vi "MetaData Channel.vi"(8 "error in (no error)":errorcluster, 11 "Node Ptr":T5 format="%.0x") -> (0 "error out":errorcluster)   [LabVIEW 2019, in "Instrument Addon System Explorer.lvlib"]
uses:
  Instrument Addon System Explorer.lvlib
  <vilib>/NI VeriStand/Custom Device API/Custom Device Item Ref.ctl
  Addon Shared/Types/Protocol Data Type.ctl
  Addon Shared/Types/Metadata Channel Type.ctl
  Addon Shared/Types/Type Cast Type.ctl
  Addon Shared/Types/Endian.ctl
  Addon Shared/Types/FG Control.ctl
  Addon Shared/SubVIs/Constants.vi
  <vilib>/NI VeriStand/Custom Device API/NI VeriStand - Get Item Property.vi
  <vilib>/NI VeriStand/Custom Device API/Get Item Property (U32).vi
  <vilib>/NI VeriStand/Custom Device API/Get Item Property (String Array).vi
  <vilib>/NI VeriStand/Custom Device API/Get Item Property (String).vi
  <vilib>/NI VeriStand/Custom Device API/NI VeriStand - Set Item Property.vi
  <vilib>/NI VeriStand/Custom Device API/Set Item Property (U32).vi
  <vilib>/NI VeriStand/Custom Device API/Set Item Property (String Array).vi
  Addon Shared/SubVIs/Set Channel Value Table.vi
  <vilib>/NI VeriStand/Custom Device API/Set Item Property (String).vi
  <vilib>/NI VeriStand/Custom Device API/Custom Device API.lvlib
  Addon Shared/Instrument Addon Shared.lvlib
  APIs/Scripting API/Instrument Addon Scripting API.lvlib
panel:
  in  "Delimiter":string=","
  in  "Reset":bool
  in  "Create":bool
  in  "Elements":u32
  in  "Units":string
  in  "Default Value":dbl
  out "Channel Type (Tab)":enum32{"List", "Format", "Type Cast"}(tab)
  in  "Remove":bool
  in  "Add":bool
  in  "Enumerated List":i32(listbox)
  in  "Test Value":dbl
  in  "Format String":string="%.3g"
  out "Validated String":string
  in  "Endian":T1=enum."Little"
  in  "Type":T2
  in  "Channel Type":T3
  out "Data Type":T4
  in  "Header 2":cluster{"Section Name":string}={"Section Name"="MetaData Format Settings"}
  in  "SHDocVw.IWebBrowser":refnum<k7>(container)
  in  "Header":cluster{"Section Name":string}={"Section Name"="MetaData Settings"}
  in  "Description":string
  in  "Name":string
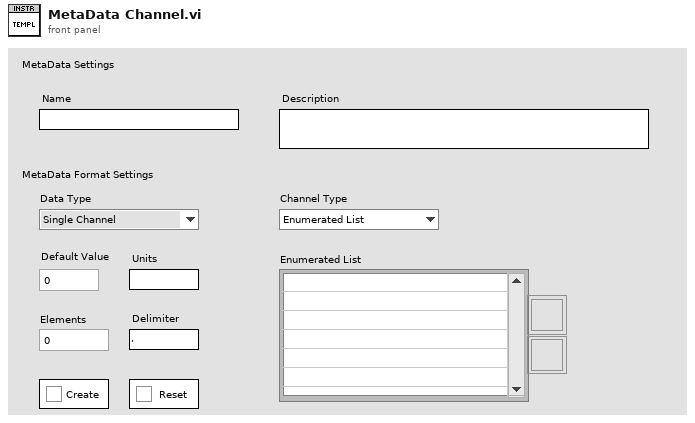
[diagram p1: front panel]
types:
  T1 = typedef "Instrument Addon Shared.lvlib/Endian.ctl" = enum16{"Native", "Little", "Big"}
  T2 = typedef "Instrument Addon Shared.lvlib/Type Cast Type.ctl" = enum16{"DBL", "SGL", "U64", "U32", "U16", "U8", "I64", "I32", "I16", "I8"}
  T3 = typedef "Instrument Addon Shared.lvlib/Metadata Channel Type.ctl" = enum16{"Enumerated List", "Format", "Type Cast"}
  T4 = typedef "Instrument Addon Shared.lvlib/Protocol Data Type.ctl" = enum16{"Single Channel", "Array"}
  T5 = typedef "Custom Device API.lvlib/Custom Device Item Ref.ctl" = u64
  T6 = typedef "Instrument Addon Shared.lvlib/FG Control.ctl" = enum16{"Get", "Set"}
  T7 = typedef "Custom Device API.lvlib/Custom Device Item Info.ctl" = cluster{"Name":string, "Is Channel":bool, "GUID":string, "Is Waveform":bool}
  T8 = typedef "Instrument Addon Shared.lvlib/MetaData Parameters.ctl" = cluster{"Data Type":T4, "Channel Type":T3, "List":string[], "Format String":string, "Type":T2, "Delimiter":string, "Endian":T1}
  T9 = typedef "Custom Device API.lvlib/Custom Device Channel.ctl" = cluster{"Type":T10, "Units":string, "Default Value":dbl, "Faultable":bool, "Scalable":bool}
  T10 = typedef "Custom Device API.lvlib/Custom Device Channel Type.ctl" = enum16{"Input", "Output"}
  T11 = typedef "Custom Device API.lvlib/Custom Device Commands.ctl" = enum16{"Default", "Item renamed", "Shutdown", "Dynamic button pressed"}
  T12 = typedef "Instrument Addon Scripting API.lvlib/Array Element.ctl" = cluster{"Name":string, "Default Value":dbl, "Units":string}
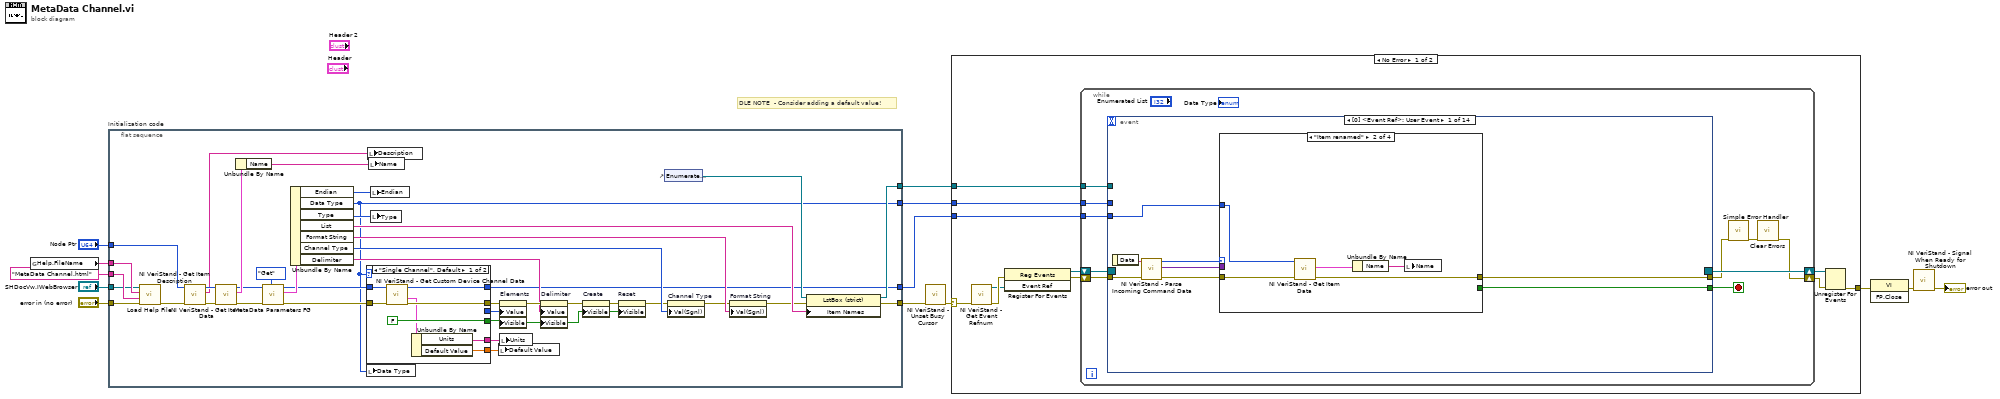
[diagram p0: block diagram]
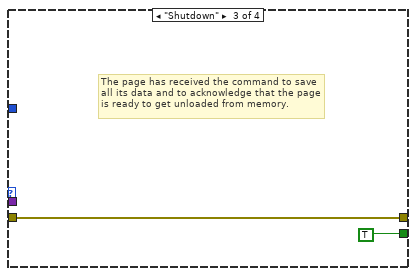
[diagram p3: hidden frame]
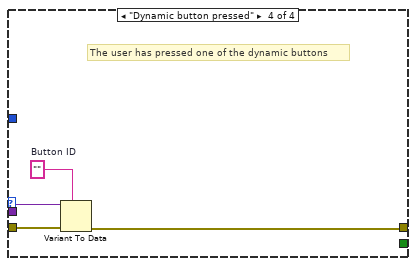
[diagram p4: hidden frame]
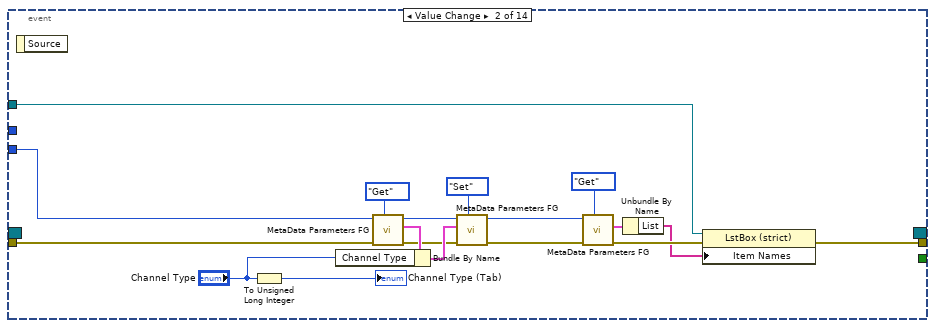
[diagram p5: hidden frame]
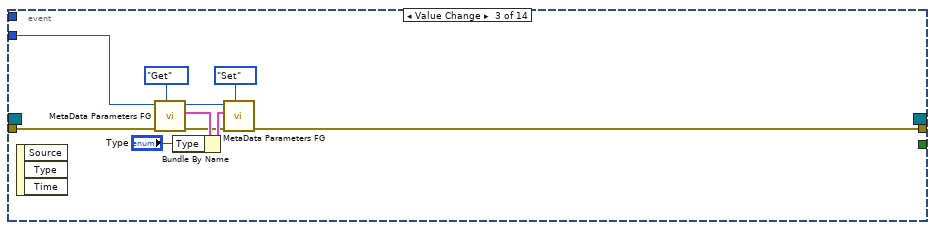
[diagram p6: hidden frame]
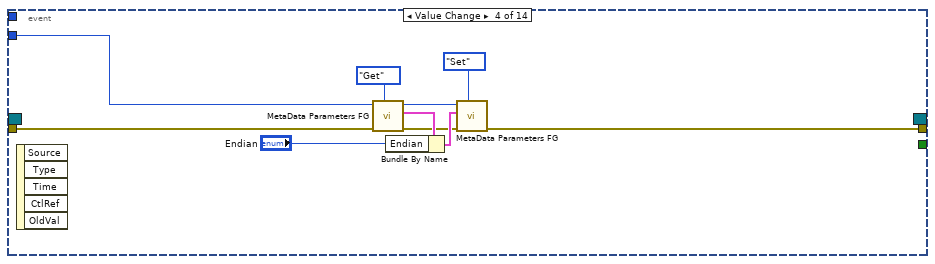
[diagram p7: hidden frame]
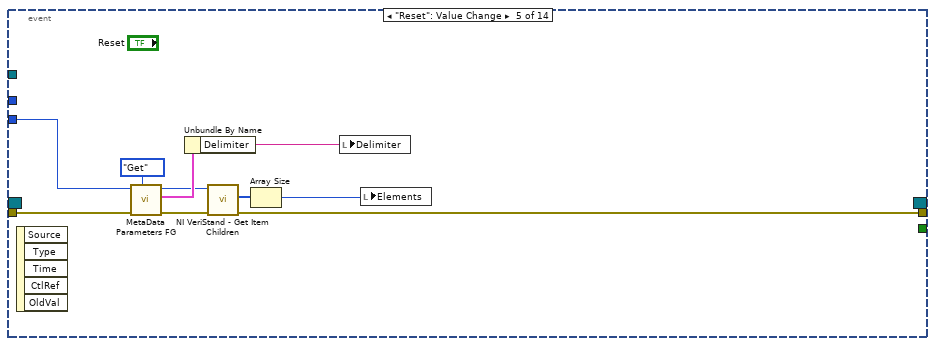
[diagram p8: hidden frame]
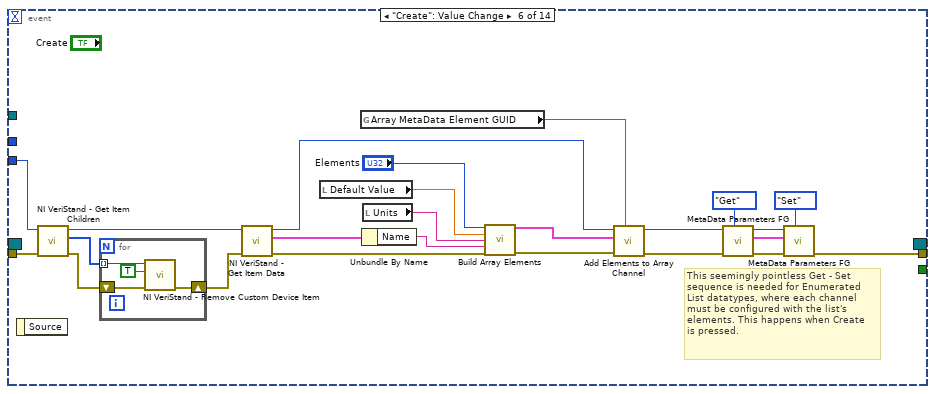
[diagram p9: hidden frame]
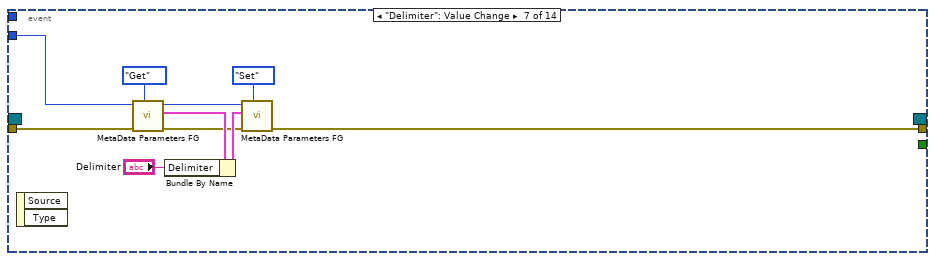
[diagram p10: hidden frame]
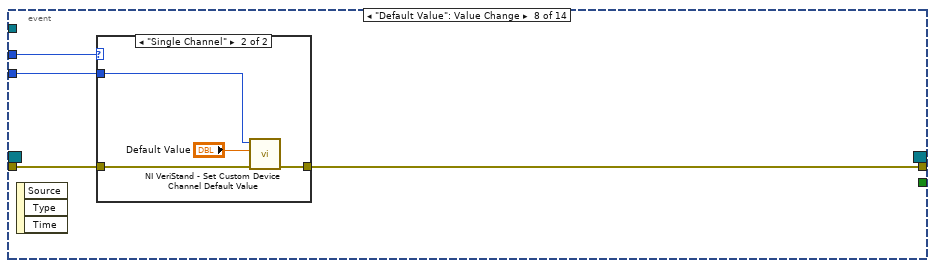
[diagram p11: hidden frame]
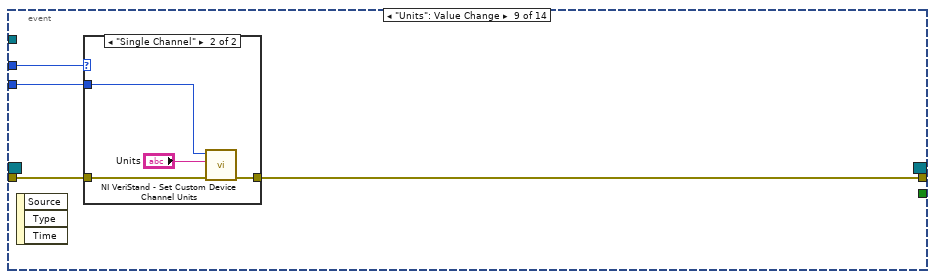
[diagram p13: hidden frame]
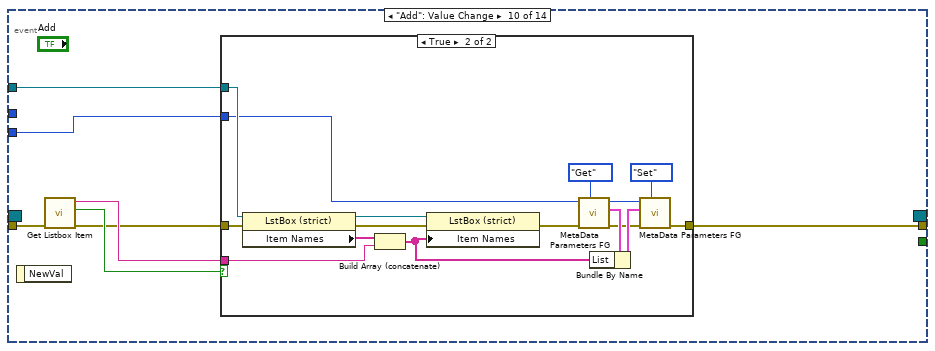
[diagram p15: hidden frame]
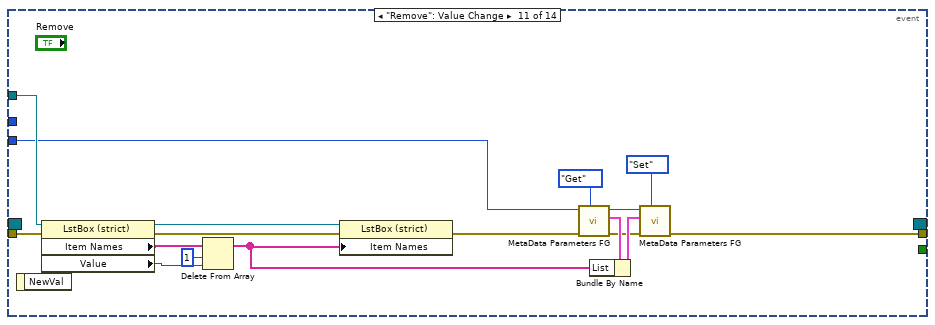
[diagram p17: hidden frame]
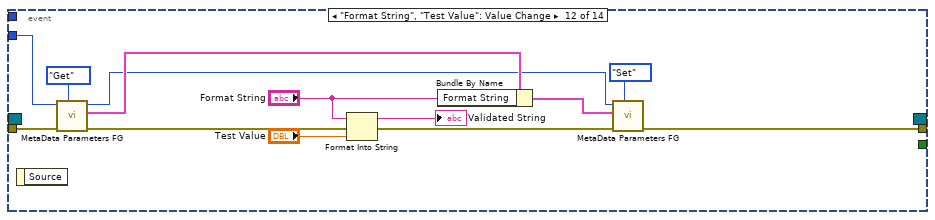
[diagram p18: hidden frame]
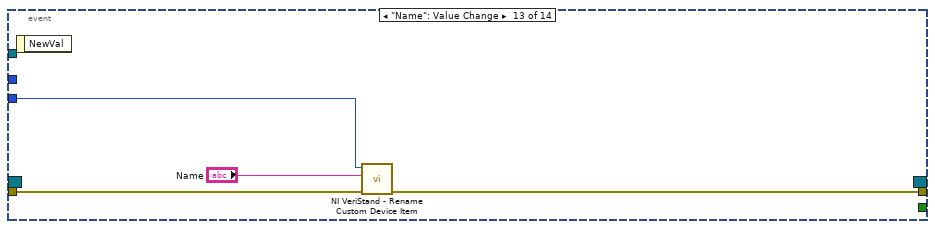
[diagram p19: hidden frame]
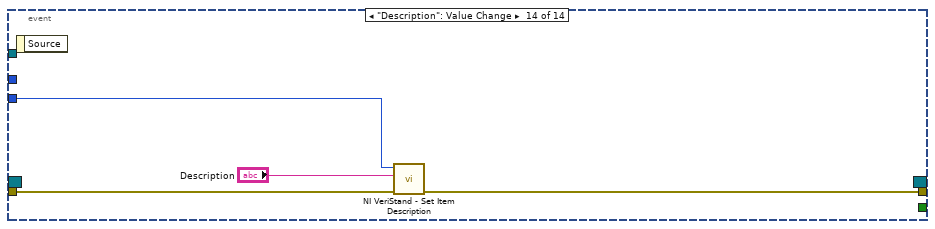
[diagram p20: hidden frame]
diagram:
  # "DLE NOTE  - Consider adding a default value!"
  n1 = global read "Constants.vi" "Help.FileName"() -> (w1:string)
  n2 = flat-sequence "Initialization code" {
    tunnel: "error in (no error)" -> [w47]
    tunnel: "Node Ptr" -> [w32]
    tunnel: [w36] -> w9
    tunnel: [w20] -> w3
    tunnel: w1 -> [w46]
    tunnel: "MetaData Channel.html" ("HTML File") -> [w45]
    tunnel: "SHDocVw.IWebBrowser" -> [w44]
    tunnel: [w34] -> w4
    tunnel: [w17] -> w2
    frame #0 {
      n3 = call "Load Help File.vi"("error in (no error)"=w47, "HTML File"=w45, "Main CHM File"=w46, "SHDocVw.IWebBrowser2"=w44) -> ("error out"=w33:errorcluster)  [unwired: 7 in]
      n4 = call <vilib>:"NI VeriStand - Get Item Description.vi"("error in (no error)"=w33, "Item Ref in"=w32) -> ("error out"=w50:errorcluster, "Description"=w51:string, "Item Ref out"=w52:T5)  [unwired: 7 out]
      n5 = call <vilib>:"NI VeriStand - Get Item Data.vi"("error in (no error)"=w50, "Item Ref in"=w52) -> ("error out"=w25:errorcluster, "Item Info"=w49:T7, "Item Ref out"=w24:T5)  [unwired: 7 out]
      n6 = Unbundle By Name(w49) -> ("Name"=w48:string)
      n7 = call "MetaData Parameters FG.vi"("Action"=FG_Control."Get", "error in (no error)"=w25, "Item Ref in"=w24) -> ("error out"=w23:errorcluster, "MetaData Parameters"=w42:T8, "Item Ref out"=w22:T5)  [unwired: 6 in]
      n8 = Unbundle By Name(w42) -> ("Endian"=w15:T1, "Data Type"=w17:T4, "Type"=w31:T2, "List"=w40:string[], "Format String"=w39:string, "Channel Type"=w41:T3, "Delimiter"=w26:string)
      n9 = local write "Data Type"(w17) -> ()
      n10 = case shown="\"Single Channel\", Default" w17 {
        tunnel: [FALSE TRUE] -> w14
        tunnel: w23 -> [w59 w64]
        tunnel: w22 -> [w58 w68]
        tunnel: [w57 w63] -> w21
        tunnel: [w56 w65] -> w20
        tunnel: [w54 ""] -> w19
        tunnel: [w53 0.0 ("Default Value")] -> w18
        tunnel: [_ w61] -> w16
        frame "Single Channel", Default {
          n11 = call <vilib>:"NI VeriStand - Get Custom Device Channel Data.vi"("error in (no error)"=w59, "Channel Ref in"=w58) -> ("error out"=w57:errorcluster, "Channel"=w55:T9, "Channel Ref out"=w56:T5)  [unwired: 4 in, 3 out]
          n12 = Unbundle By Name(w55) -> ("Units"=w54:string, "Default Value"=w53:dbl)
        }
        frame "Array" {
          n13 = call <vilib>:"NI VeriStand - Get Item Children.vi"("error in (no error)"=w64, "Item Ref in"=w68) -> ("error out"=w63:errorcluster, "Child Refs"=w62:T5[], "Item Ref out"=w65:T5)  [unwired: 6 in, 1 out]
          n14 = Array Size(array=w62) -> (size(s)=w61:i32)
        }
      }
      n15 = local write "Description"(w51) -> ()
      n16 = local write "Name"(w48) -> ()
      n17 = local write "Endian"(w15) -> ()
      n18 = local write "Type"(w31) -> ()
      n19 = local write "Default Value"(w18) -> ()
      n20 = property on="Elements" class="DigNum (strict)"(error in=w21, "Value"=w16, "Visible"=w14) -> (error out=w28:errorcluster)  [unwired: 1 in, 1 out]
      n21 = local write "Units"(w19) -> ()
      n22 = property on="Delimiter" class="Str"(error in=w28, "Value"=w26, "Visible"=w14) -> (error out=w29:errorcluster)  [unwired: 1 in, 1 out]
      n23 = property on="Create" class="Bool"(error in=w29, "Visible"=w14) -> (error out=w30:errorcluster)  [unwired: 1 in, 1 out]
      n24 = property on="Reset" class="Bool"(error in=w30, "Visible"=w14) -> (error out=w27:errorcluster)  [unwired: 1 in, 1 out]
      n25 = control-ref of="Enumerated List"() -> (w35:refnum<vi>)
      n26 = property on="Channel Type" class="Enum (strict)"(error in=w27, "Val(Sgnl)"=w41) -> (error out=w38:errorcluster)  [unwired: 1 in, 1 out]
      n27 = property on="Format String" class="Str"(error in=w38, "Val(Sgnl)"=w39) -> (error out=w37:errorcluster)  [unwired: 1 in, 1 out]
      n28 = property class="LstBox (strict)"(reference=w35, error in=w37, "Item Names"=w40) -> (reference out=w34:refnum<vi>, error out=w36:errorcluster)
    }
  }
  n29 = call <vilib>:"NI VeriStand - Unset Busy Cursor.vi"("error in (no error)"=w9) -> ("error out"=w8:errorcluster)  [unwired: 10 out]
  n30 = case shown="No Error" w8 {
    selector: w8 -> [w72 w279]
    tunnel: [w77 w277] -> w13
    tunnel: w3 -> [w73 _]
    tunnel: w4 -> [w71 _]
    tunnel: w2 -> [w70 _]
    frame No Error {
      n31 = call <vilib>:"NI VeriStand - Get Event Refnum.vi"("error in (no error)"=w72) -> ("error out"=w80:errorcluster, "Event Ref"=w76:refnum<user-event>)  [unwired: 9 out]
      n32 = register-events(error in=w80, w76) -> (reference out=w74:refnum<event-registration>, error out=w75:errorcluster)  [unwired: 1 in]
      n33 = while {
        tunnel: w73 -> [w86]
        shift-right: [w83] -> w78
        shift-left: w75 -> [w89]
        shift-right: [w90] -> w79
        shift-left: w74 -> [w88]
        tunnel: w71 -> [w82]
        tunnel: w70 -> [w81]
        stop <- w87 stop-if-true
        n34 = event shown="[0] <Event Ref>: User Event" {
          selector: w88 -> [_ _ _ _ _ _ _ _ _ _ _ _ _ _]
          dyn-events: [_ _ _ _ _ _ _ _ _ _ _ _ _ _] -> w90
          timeout: _ -> [_ _ _ _ _ _ _ _ _ _ _ _ _ _]
          tunnel: w89 -> [w98 w122 w133 w143 w156 w178 w189 w200 w209 w216 w252 w264 w272 w275]
          tunnel: [w94 _ _ _ _ _ _ _ _ _ _ _ _ _] -> w87
          tunnel: [w93 w111 w129 w140 w150 w169 w187 w199 w208 w220 w241 w265 w271 w274] -> w85
          tunnel: w86 -> [w92 w121 w132 w142 w155 w181 w188 w198 w207 w219 w239 w262 w270 w276]
          tunnel: w82 -> [_ w113 _ _ _ _ _ _ _ w221 w255 _ _ _]
          tunnel: w81 -> [_ _ _ _ _ _ _ w197 w206 _ _ _ _ _]
          event User Event {
            n35 = event-data() -> ("Data"=w97:string)  [unwired: 1 out]
            n36 = call <vilib>:"NI VeriStand - Parse Incoming Command Data.vi"("error in (no error)"=w98, "Incoming data"=w97) -> ("error out"=w96:errorcluster, "Outgoing data"=w91:variant, "Action"=w95:T11)  [unwired: 7 out]
            n37 = case shown="\"Item renamed\"" w95 {
              tunnel: w96 -> [w99 w104 w105 w110]
              tunnel: [_ _ TRUE _] -> w94
              tunnel: [w99 w101 w105 w107] -> w93
              tunnel: w92 -> [_ w103 _ _]
              tunnel: w91 -> [_ _ _ w109]
              frame "Default", Default {
              }
              frame "Item renamed" {
                n38 = call <vilib>:"NI VeriStand - Get Item Data.vi"("error in (no error)"=w104, "Item Ref in"=w103) -> ("error out"=w101:errorcluster, "Item Info"=w102:T7)  [unwired: 8 out]
                n39 = Unbundle By Name(w102) -> ("Name"=w100:string)
                n40 = local write "Name"(w100) -> ()
              }
              frame "Shutdown" {
                # "The page has received the command to save all its data and to acknowledge that the page is ready to get unloaded from memory."
              }
              frame "Dynamic button pressed" {
                w108 = ""  # Button ID
                # "The user has pressed one of the dynamic buttons"
                n41 = Variant To Data(error in=w110, type=w108, Variant=w109) -> (error out=w107:errorcluster)  [unwired: 1 out]
              }
            }
          }
          event Value Change {
            n42 = event-data() -> ()  [unwired: 2 out]
            n43 = To Unsigned Long Integer(number="Channel Type") -> (unsigned 32bit integer=→"Channel Type (Tab)":u32)
            n44 = call "MetaData Parameters FG.vi"("Action"=FG_Control."Get", "error in (no error)"=w122, "Item Ref in"=w121) -> ("error out"=w120:errorcluster, "MetaData Parameters"=w126:T8, "Item Ref out"=w124:T5)  [unwired: 6 in]
            n45 = Bundle By Name(cluster=w126, "Channel Type"="Channel Type") -> (w125:T8)
            n46 = call "MetaData Parameters FG.vi"("Action"=FG_Control."Set", "error in (no error)"=w120, "MetaData Parameters"=w125, "Item Ref in"=w124) -> ("error out"=w115:errorcluster, "Item Ref out"=w114:T5)  [unwired: 5 in, 1 out]
            n47 = call "MetaData Parameters FG.vi"("Action"=FG_Control."Get", "error in (no error)"=w115, "Item Ref in"=w114) -> ("error out"=w117:errorcluster, "MetaData Parameters"=w118:T8)  [unwired: 6 in, 1 out]
            n48 = Unbundle By Name(w118) -> ("List"=w116:string[])
            n49 = property class="LstBox (strict)"(reference=w113, error in=w117, "Item Names"=w116) -> (error out=w111:errorcluster)  [unwired: 1 out]
          }
          event Value Change {
            n50 = event-data() -> ()  [unwired: 4 out]
            n51 = call "MetaData Parameters FG.vi"("Action"=FG_Control."Get", "error in (no error)"=w133, "Item Ref in"=w132) -> ("error out"=w131:errorcluster, "MetaData Parameters"=w137:T8, "Item Ref out"=w135:T5)  [unwired: 6 in]
            n52 = Bundle By Name(cluster=w137, "Type"="Type") -> (w136:T8)
            n53 = call "MetaData Parameters FG.vi"("Action"=FG_Control."Set", "error in (no error)"=w131, "MetaData Parameters"=w136, "Item Ref in"=w135) -> ("error out"=w129:errorcluster)  [unwired: 5 in, 2 out]
          }
          event Value Change {
            n54 = event-data() -> ()  [unwired: 6 out]
            n55 = call "MetaData Parameters FG.vi"("Action"=FG_Control."Get", "error in (no error)"=w143, "Item Ref in"=w142) -> ("error out"=w141:errorcluster, "MetaData Parameters"=w147:T8, "Item Ref out"=w145:T5)  [unwired: 6 in]
            n56 = Bundle By Name(cluster=w147, "Endian"="Endian") -> (w146:T8)
            n57 = call "MetaData Parameters FG.vi"("Action"=FG_Control."Set", "error in (no error)"=w141, "MetaData Parameters"=w146, "Item Ref in"=w145) -> ("error out"=w140:errorcluster)  [unwired: 5 in, 2 out]
          }
          event "Reset": Value Change {
            n58 = event-data() -> ()  [unwired: 6 out]
            n59 = call "MetaData Parameters FG.vi"("Action"=FG_Control."Get", "error in (no error)"=w156, "Item Ref in"=w155) -> ("error out"=w151:errorcluster, "MetaData Parameters"=w158:T8, "Item Ref out"=w152:T5)  [unwired: 6 in]
            n60 = Unbundle By Name(w158) -> ("Delimiter"=w154:string)
            n61 = call <vilib>:"NI VeriStand - Get Item Children.vi"("error in (no error)"=w151, "Item Ref in"=w152) -> ("error out"=w150:errorcluster, "Child Refs"=w153:T5[])  [unwired: 6 in, 2 out]
            n62 = Array Size(array=w153) -> (size(s)=w149:i32)
            n63 = local write "Delimiter"(w154) -> ()
            n64 = local write "Elements"(w149) -> ()
          }
          event "Create": Value Change {
            # "This seemingly pointless Get - Set\nsequence is needed for Enumerated\nList datatypes, where each channel\nmust be configured with the list's\nelements. This happens when Create\nis pressed."
            n65 = event-data() -> ()  [unwired: 2 out]
            n66 = call <vilib>:"NI VeriStand - Get Item Children.vi"("error in (no error)"=w178, "Item Ref in"=w181) -> ("error out"=w175:errorcluster, "Child Refs"=w176:T5[], "Item Ref out"=w179:T5)  [unwired: 6 in, 1 out]
            n67 = for {
              shift-right: [w185] -> w177
              shift-left: w175 -> [w183]
              tunnel: w176 -> [w184] mode=indexing
              n68 = call <vilib>:"NI VeriStand - Remove Custom Device Item.vi"("error in (no error)"=w183, "Force Delete (F)"=TRUE, "Item Ref in"=w184) -> ("error out"=w185:errorcluster)  [unwired: 7 in, 1 out]
            }
            n69 = call <vilib>:"NI VeriStand - Get Item Data.vi"("error in (no error)"=w177, "Item Ref in"=w179) -> ("error out"=w180:errorcluster, "Item Info"=w182:T7, "Item Ref out"=w164:T5)  [unwired: 7 out]
            n70 = local read "Default Value"() -> (w166:dbl)
            n71 = global read "Constants.vi" "Array MetaData Element GUID"() -> (w159:string)
            n72 = Unbundle By Name(w182) -> ("Name"=w168:string)
            n73 = local read "Units"() -> (w167:string)
            n74 = call "Build Array Elements.vi"("Elements"="Elements", "Default Value"=w166, "Units"=w167, "Name"=w168, "error in (no error)"=w180) -> ("Array"=w163:T12[], "error out"=w162:errorcluster)  [unwired: 9 in]
            n75 = call "Add Elements to Array Channel.vi"("array element GUID"=w159, "error in (no error)"=w162, "array elements"=w163, "array refnum in"=w164) -> ("error out"=w161:errorcluster, "array refnum out"=w160:T5)  [unwired: 5 in, 1 out]
            n76 = call "MetaData Parameters FG.vi"("Action"=FG_Control."Get", "error in (no error)"=w161, "Item Ref in"=w160) -> ("error out"=w171:errorcluster, "MetaData Parameters"=w170:T8, "Item Ref out"=w173:T5)  [unwired: 6 in]
            n77 = call "MetaData Parameters FG.vi"("Action"=FG_Control."Set", "error in (no error)"=w171, "MetaData Parameters"=w170, "Item Ref in"=w173) -> ("error out"=w169:errorcluster)  [unwired: 5 in, 2 out]
          }
          event "Delimiter": Value Change {
            n78 = event-data() -> ()  [unwired: 3 out]
            n79 = call "MetaData Parameters FG.vi"("Action"=FG_Control."Get", "error in (no error)"=w189, "Item Ref in"=w188) -> ("error out"=w192:errorcluster, "MetaData Parameters"=w196:T8, "Item Ref out"=w194:T5)  [unwired: 6 in]
            n80 = Bundle By Name(cluster=w196, "Delimiter"="Delimiter") -> (w195:T8)
            n81 = call "MetaData Parameters FG.vi"("Action"=FG_Control."Set", "error in (no error)"=w192, "MetaData Parameters"=w195, "Item Ref in"=w194) -> ("error out"=w187:errorcluster)  [unwired: 5 in, 2 out]
          }
          event "Default Value": Value Change {
            n82 = event-data() -> ()  [unwired: 4 out]
            n83 = case shown="\"Single Channel\"" w197 {
              tunnel: w200 -> [w201 w205]
              tunnel: [w201 w204] -> w199
              tunnel: w198 -> [_ w203]
              frame "Array" {
              }
              frame "Single Channel" {
                n84 = call <vilib>:"NI VeriStand - Set Custom Device Channel Default Value.vi"("error in (no error)"=w205, "Default Value"="Default Value", "Channel Ref in"=w203) -> ("error out"=w204:errorcluster)  [unwired: 7 in, 1 out]
              }
            }
          }
          event "Units": Value Change {
            n85 = event-data() -> ()  [unwired: 4 out]
            n86 = case shown="\"Single Channel\"" w206 {
              tunnel: w209 -> [w210 w214]
              tunnel: [w210 w213] -> w208
              tunnel: w207 -> [_ w212]
              frame "Array" {
              }
              frame "Single Channel" {
                n87 = call <vilib>:"NI VeriStand - Set Custom Device Channel Units.vi"("error in (no error)"=w214, "Units"="Units", "Channel Ref in"=w212) -> ("error out"=w213:errorcluster)  [unwired: 7 in, 1 out]
              }
            }
          }
          event "Add": Value Change {
            n88 = event-data() -> ()  [unwired: 2 out]
            n89 = call "Get Listbox Item.vi"("error in (no error)"=w216) -> ("error out"=w215:errorcluster, "OK?"=w217:bool, "Item out"=w218:string)  [unwired: 8 in]
            n90 = case shown="True" w217 {
              tunnel: w221 -> [_ w238]
              tunnel: w215 -> [w222 w237]
              tunnel: w218 -> [_ w233]
              tunnel: [w222 w224] -> w220
              tunnel: w219 -> [_ w226]
              frame False {
              }
              frame True {
                n91 = property class="LstBox (strict)"(reference=w238, error in=w237) -> (reference out=w236:refnum<vi>, error out=w235:errorcluster, "Item Names"=w234:string[])
                n92 = Build Array (concatenate)(w234, w233) -> (w223:string[])
                n93 = property class="LstBox (strict)"(reference=w236, error in=w235, "Item Names"=w223) -> (error out=w225:errorcluster)  [unwired: 1 out]
                n94 = call "MetaData Parameters FG.vi"("Action"=FG_Control."Get", "error in (no error)"=w225, "Item Ref in"=w226) -> ("error out"=w227:errorcluster, "MetaData Parameters"=w231:T8, "Item Ref out"=w229:T5)  [unwired: 6 in]
                n95 = Bundle By Name(cluster=w231, "List"=w223) -> (w230:T8)
                n96 = call "MetaData Parameters FG.vi"("Action"=FG_Control."Set", "error in (no error)"=w227, "MetaData Parameters"=w230, "Item Ref in"=w229) -> ("error out"=w224:errorcluster)  [unwired: 5 in, 2 out]
              }
            }
          }
          event "Remove": Value Change {
            n97 = event-data() -> ()  [unwired: 2 out]
            n98 = property class="LstBox (strict)"(reference=w255, error in=w252) -> (reference out=w254:refnum<vi>, error out=w253:errorcluster, "Item Names"=w251:string[], "Value"=w250:i32)
            n99 = Delete From Array(array=w251, length=1, index=w250) -> (array with subset deleted=w240:string[])  [unwired: 1 out]
            n100 = property class="LstBox (strict)"(reference=w254, error in=w253, "Item Names"=w240) -> (error out=w242:errorcluster)  [unwired: 1 out]
            n101 = call "MetaData Parameters FG.vi"("Action"=FG_Control."Get", "error in (no error)"=w242, "Item Ref in"=w239) -> ("error out"=w243:errorcluster, "MetaData Parameters"=w247:T8, "Item Ref out"=w245:T5)  [unwired: 6 in]
            n102 = Bundle By Name(cluster=w247, "List"=w240) -> (w246:T8)
            n103 = call "MetaData Parameters FG.vi"("Action"=FG_Control."Set", "error in (no error)"=w243, "MetaData Parameters"=w246, "Item Ref in"=w245) -> ("error out"=w241:errorcluster)  [unwired: 5 in, 2 out]
          }
          event "Format String", "Test Value": Value Change {
            n104 = event-data() -> ()  [unwired: 2 out]
            n105 = call "MetaData Parameters FG.vi"("Action"=FG_Control."Get", "error in (no error)"=w264, "Item Ref in"=w262) -> ("error out"=w263:errorcluster, "MetaData Parameters"=w260:T8, "Item Ref out"=w257:T5)  [unwired: 6 in]
            n106 = Format Into String(format string="Format String", error in=w263, "Test Value") -> (resulting string=→"Validated String":string, error out=w266:errorcluster)  [unwired: 1 in]
            n107 = Bundle By Name(cluster=w260, "Format String"="Format String") -> (w258:T8)
            n108 = call "MetaData Parameters FG.vi"("Action"=FG_Control."Set", "error in (no error)"=w266, "MetaData Parameters"=w258, "Item Ref in"=w257) -> ("error out"=w265:errorcluster)  [unwired: 5 in, 2 out]
          }
          event "Name": Value Change {
            n109 = event-data() -> ()  [unwired: 2 out]
            n110 = call <vilib>:"NI VeriStand - Rename Custom Device Item.vi"("error in (no error)"=w272, "New Name"="Name", "Item Ref in"=w270) -> ("error out"=w271:errorcluster)  [unwired: 1 in, 7 out]
          }
          event "Description": Value Change {
            n111 = event-data() -> ()  [unwired: 2 out]
            n112 = call <vilib>:"NI VeriStand - Set Item Description.vi"("error in (no error)"=w275, "Description"="Description", "Item Ref in"=w276) -> ("error out"=w274:errorcluster)  [unwired: 8 out]
          }
        }
        n113 = call <vilib>:"Simple Error Handler.vi"("error in (no error)"=w85) -> ("error out"=w84:errorcluster)  [unwired: 1 in, 7 out]
        n114 = call <vilib>:"Clear Errors.vi"("error in (no error)"=w84) -> ("error out"=w83:errorcluster)  [unwired: 1 in, 5 out]
      }
      n115 = Unregister For Events(event registration refnum=w79, error in=w78) -> (error out=w77:errorcluster)
    }
    frame Error {
      n116 = call <vilib>:"Simple Error Handler.vi"("error in (no error)"=w279) -> ("error out"=w278:errorcluster)  [unwired: 1 in, 7 out]
      n117 = call <vilib>:"Clear Errors.vi"("error in (no error)"=w278) -> ("error out"=w277:errorcluster)  [unwired: 1 in, 5 out]
    }
  }
  n118 = invoke class="VI" method="FP.Close"(error in=w13) -> (error out=w12:errorcluster)  [unwired: 2 in, 2 out]
  n119 = call <vilib>:"NI VeriStand - Signal When Ready for Shutdown.vi"("error in (no error)"=w12) -> ("error out"=→"error out":errorcluster)  [unwired: 10 out]
